vi "GUILaptop.vi"() -> ()   [LabVIEW 2016]
uses:
  Control/Fahrart.ctl
  Control/GUICluster.ctl
panel:
  out "Leistung Chart":dbl(graph)
  out "Drehzahl Chart":dbl(graph)
  out "Drehzahl":dbl=6.577122973792136
  out "hinten links":dbl(slide) scale=0.0..150.0
  out "hinten rechts":dbl(slide) scale=0.0..150.0
  in  "stop":bool
  out "Leistung":dbl=6.577122973792136
  in  "Fahrzustand":T1
  out "PID gains out":T2
  out "rechts":dbl(slide) scale=0.0..150.0
  out "links":dbl(slide) scale=0.0..150.0
  out "schräg L":dbl(slide) scale=0.0..150.0
  out "schräge R":dbl(slide) scale=0.0..150.0
  out "gerade L":dbl(slide) scale=0.0..150.0
  out "gerade R":dbl(slide) scale=0.0..150.0
  out "Rundenzeiten":T3
  out "Linefollow_Array":bool[](array[boolean])
  in  "Geschwindigkeit multiplikator":dbl(knob)=0.039196582802747515 scale=0.0..1.0
  # "Minimum"
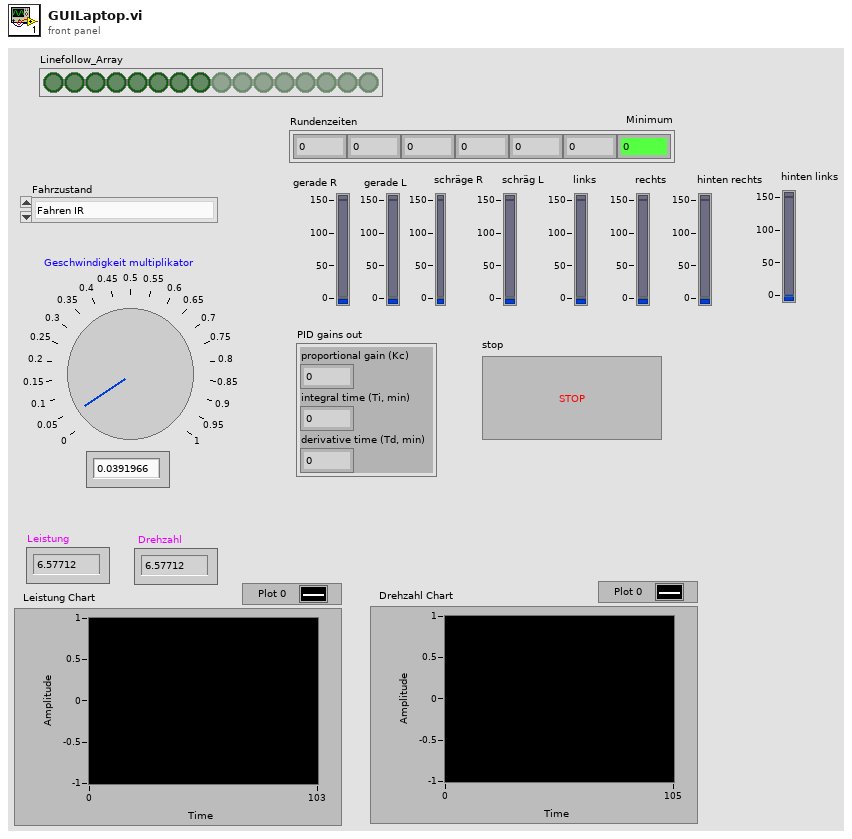
[diagram p1: front panel]
types:
  T1 = typedef "Fahrart.ctl" = enum16{"Fahren IR", "Fahren Array", "Folgen", "Überholen"}
  T2 = cluster{"proportional gain (Kc)":dbl, "integral time (Ti, min)":dbl, "derivative time (Td, min)":dbl}
  T3 = cluster{"Rundenzeiten[0]":dbl, "Rundenzeiten[1]":dbl, "Rundenzeiten[2]":dbl, "Rundenzeiten[3]":dbl, "Rundenzeiten[4]":dbl, "Rundenzeiten[5]":dbl, "Rundenzeiten[8]":dbl}
  T4 = cluster{"Fahrzustand":T1, "Geschwindigkeit multiplikator":dbl, "stop":bool}
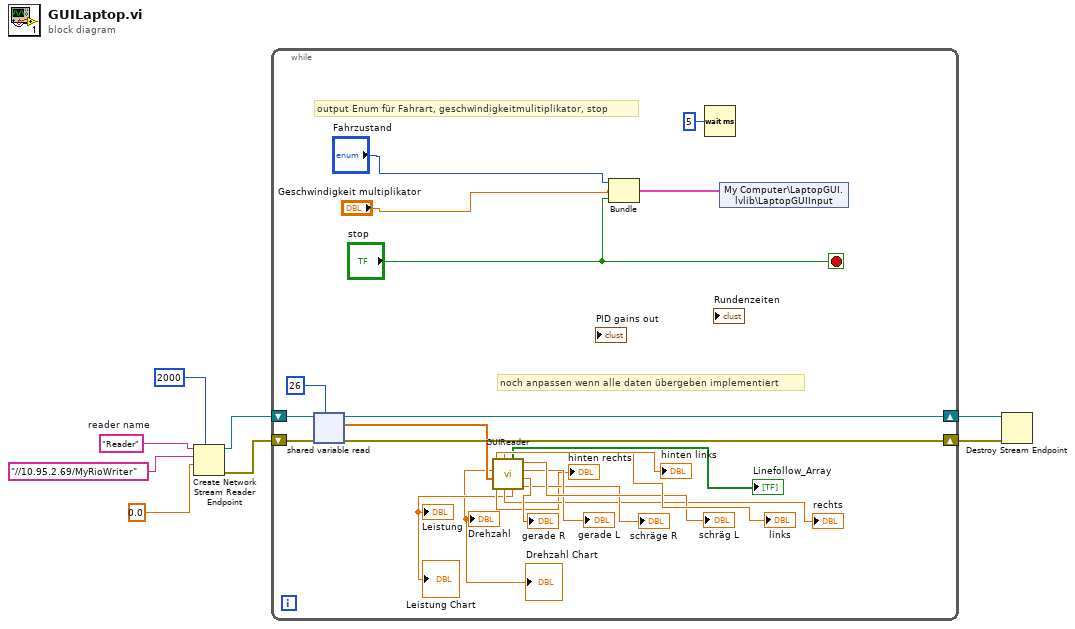
[diagram p0: block diagram]
diagram:
  w4 = "Reader"  # reader name
  n1 = Create Network Stream Reader Endpoint(7:2000 ("reader buffer size"), 9:0.0, 10:"//10.95.2.69/MyRioWriter" ("writer url"), 11:w4) -> (0:w7:errorcluster, 3:w8:refnum<k21>)  [unwired: 3 in]
  n2 = while {
    shift-right: [w28] -> w6
    shift-left: w8 -> [w30]
    shift-right: [w27] -> w5
    shift-left: w7 -> [w29]
    stop <- "stop" stop-if-true
    # "output Enum für Fahrart, geschwindigkeitmulitiplikator, stop"
    # "noch anpassen wenn alle daten übergeben implementiert"
    n3 = shared-variable-read(w30, w29, 26 ("# elements")) -> (w28:refnum<k21>, w27:errorcluster, w20:dbl[])  [unwired: 1 in, 1 out]
    n4 = call "GUIReader.vi"("Input Array"=w20) -> ("Schräg R"=→"schräge R":dbl, "gerade R"=→"gerade R":dbl, "gerade L"=→"gerade L":dbl, "Schräg L"=→"schräg L":dbl, "Leistung"=→"Leistung" →"Leistung Chart":dbl, "Linefollow_Array"=→"Linefollow_Array":bool[], "Rechts"=→"rechts":dbl, "Links"=→"links":dbl, "Hinten R"=→"hinten rechts":dbl, "Drehzahl"=→"Drehzahl" →"Drehzahl Chart":dbl, "hinten LI"=→"hinten links":dbl)
    n5 = Bundle("Fahrzustand"="Fahrzustand", "Geschwindigkeit multiplikator"="Geschwindigkeit multiplikator", "stop"="stop") -> (w23:T4)  [unwired: 1 in]
    n6 = Wait (ms)(milliseconds to wait=u32 5) -> ()  [unwired: 1 out]
    n7 = shared-variable "My Computer\\LaptopGUI.lvlib\\LaptopGUIInput"(w23) -> ()  [unwired: 1 in, 1 out]
  }
  n8 = Destroy Stream Endpoint(8:w5, 11:w6) -> ()  [unwired: 1 out]
